vi "Npsv pc test.vi"() -> ()   [LabVIEW 2017]
uses:
  MsgTypeDef.ctl
  <vilib>/WPC Systems Ltd/GECO Driver/Lib/GECOMotion/GECOMotion/_typedefine/Axis Select.ctl
  <vilib>/WPC Systems Ltd/GECO Driver/Lib/GECOMotion/GECOMotion/GECO Motion.lvclass
  <vilib>/WPC Systems Ltd/GECO Driver/Lib/GECOBase/GECO_Driver Class/Motion/_typedefine/GECO_ActiveHighLow.ctl
  <vilib>/WPC Systems Ltd/GECO Driver/Lib/GECOBase/GECO_Driver Class/GECO_Driver.lvclass
  <vilib>/WPC Systems Ltd/GECO Driver/Lib/GECOBase/GECO_Driver Class/Motion/_typedefine/GECO_Motion Operation Mode.ctl
  <vilib>/WPC Systems Ltd/GECO Driver/Lib/GECOBase/GECO_Driver Class/GECO_SlotName.ctl
  <vilib>/WPC Systems Ltd/GECO Driver/Lib/GECOBase/GECO_Driver Class/Motion/_typedefine/GECO_Stepper Output Configuration.ctl
  <vilib>/NI/Modbus Library/API/Modbus API.lvclass
  DataDef.ctl
  GyroDef.ctl
  <vilib>/Instr/_visa.llb/VISA Configure Serial Port (Instr).vi
  Reverse Polarity.ctl
  Forward Polarity.ctl
  Motion Controller Slot.ctl
  Stepper Output Configuration.ctl
  Axis Select.ctl
panel:
  out "RT Program Period":u32
  out "error IO 2":errorcluster
  out "error IO":errorcluster
  out "實際角度":cluster{"A":dbl, "B":dbl}={"A"=-3.299667554384925, "B"=3.520332445615068}
  out "實際角度Chart":cluster{"X":dbl, "Y":dbl}(graph)={"X"=-3.299667554384925, "Y"=3.520332445615068} caption="Waveform Chart - dark"
  out "Gyro\nPeriod":u32
  in  "Main Setting Tab":T1(tab)
  in  "TimerON":bool
  in  "Timer(ms)":i32=1
  in  "Serial Port":refnum<visa-resource-name>="COM3"
  in  "TCP slave port":u32=1
  in  "baud rate":u32=115200
  in  "Byte bits":u32=8
  in  "Modbus Address Starting":u32
  in  "Modbus Number of Inputs":u32=10000
  in  "Resource Name":tag="rio://192.168.0.224/RIO0"
  in  "Servo on":bool
  in  "Axis Select":T2
  in  "Stepper Output Configuration":T3=enum."CW/CCW(Two Pulse)"
  in  "Forward Enable?":bool=TRUE
  in  "Reverse Enable?":bool=TRUE
  in  "Motion Operation Mode":T4(ring)=enum."Velocity"
  in  "Forward Polarity":T5
  in  "Reverse Polarity":T6
  in  "Motion Controller Slot":T7
  in  "Target Position (0)":dbl=10000.0
  in  "Acceleration (100000)":u32=300000
  in  "Velocity (10000)":dbl=100000.0
  in  "Deacceleration (100000)":u32=300000
  in  "PID gains setting Tab":enum32{"Axis 1", "Axis 2", "Axis 3"}(tab)
  in  "PID gains":T8={"proportional gain (Kc)"=0.75, "integral time (Ti, min)"=0.01, "derivative time (Td, min)"=0.0} {"derivative time (Td, min)" format="%#_3f"; "integral time (Ti, min)" format="%#_3f"; "proportional gain (Kc)" format="%#_3f"}
  in  "PID gains 2":T8={"proportional gain (Kc)"=0.75, "integral time (Ti, min)"=0.01, "derivative time (Td, min)"=0.0} {"derivative time (Td, min)" format="%#_3f"; "integral time (Ti, min)" format="%#_3f"; "proportional gain (Kc)" format="%#_3f"}
  in  "PID gains 3":T8={"proportional gain (Kc)"=0.75, "integral time (Ti, min)"=0.01, "derivative time (Td, min)"=0.0} {"derivative time (Td, min)" format="%#_3f"; "integral time (Ti, min)" format="%#_3f"; "proportional gain (Kc)" format="%#_3f"}
  in  "ZABStop":bool
  in  "B":i32
  in  "A":i32
  in  "Z":i32=50
  in  "ZAB Start":bool
  in  "Move Setting":T9
  out "Axis 1":T10
  out "Axis 2":T10
  out "Axis 3":T10
  out "Program Period":u32
  in  "ServoButtonControl":T11
  in  "Connect":bool
  in  "Close":bool
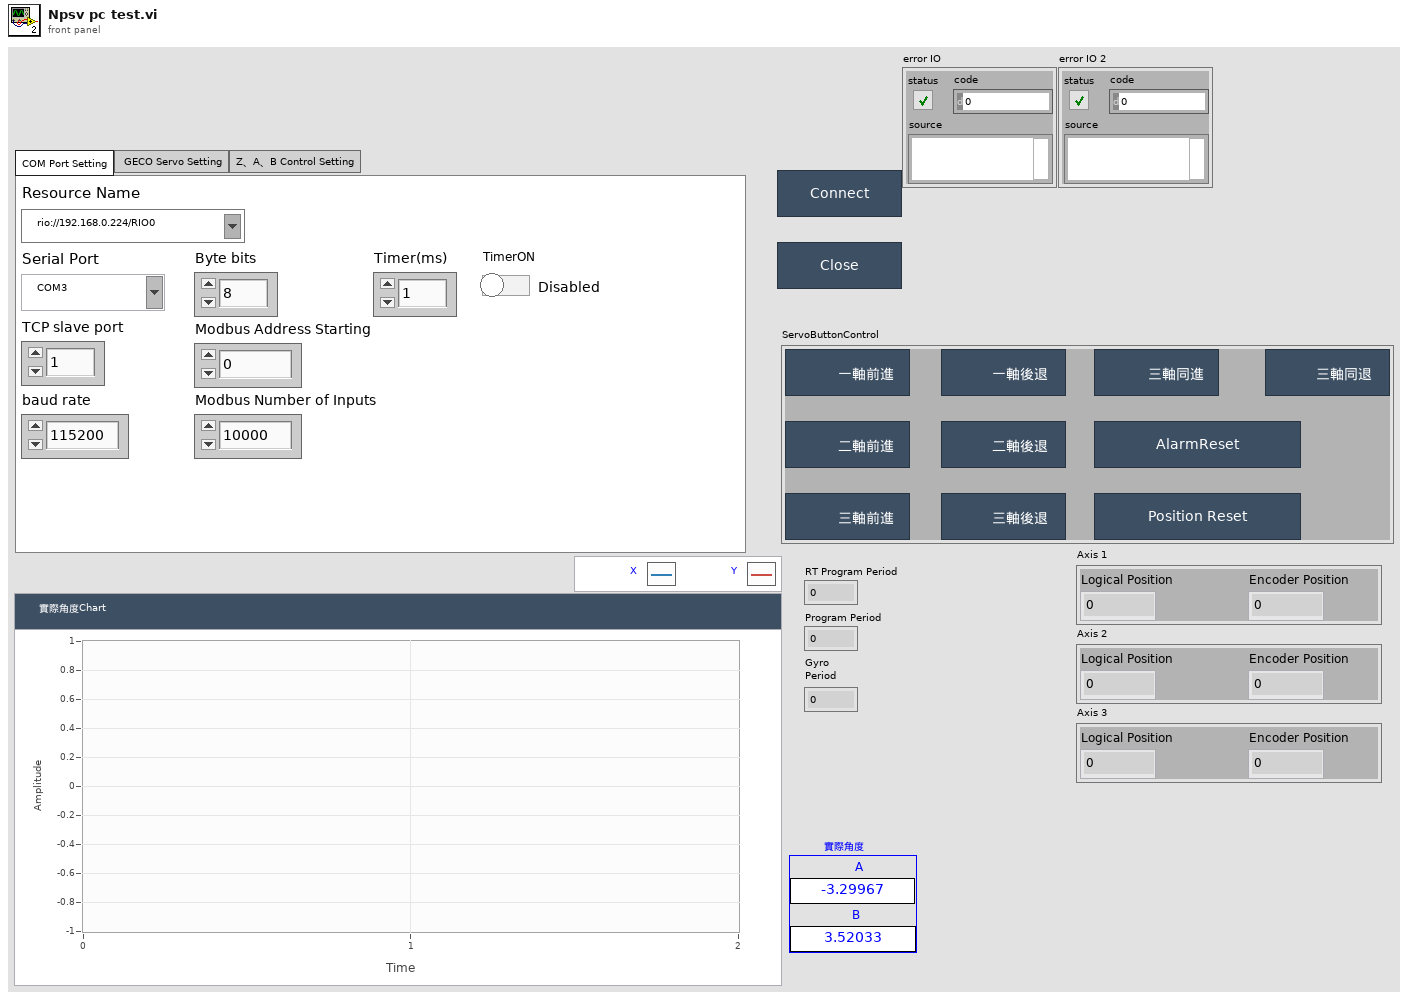
[diagram p1: front panel]
types:
  T1 = enum32{"COM Port Setting", " GECO Servo Setting", "Z、A、B Control Setting"}
  T2 = typedef "Axis Select.ctl" = enum16{"Axis 1", "Axis 2", "Axis 3", "Axis 4"}
  T3 = typedef "Stepper Output Configuration.ctl" = enum16{"Step/Dir(One Pulse)", "CW/CCW(Two Pulse)"}
  T4 = enum16{"Absolute Position", "Relative Position", "Velocity"}
  T5 = typedef "Forward Polarity.ctl" = enum16{"Active High", "Active Low"}
  T6 = typedef "Reverse Polarity.ctl" = enum16{"Active High", "Active Low"}
  T7 = typedef "Motion Controller Slot.ctl" = enum16{"C1", "C2", "C3", "C4"}
  T8 = cluster{"proportional gain (Kc)":dbl, "integral time (Ti, min)":dbl, "derivative time (Td, min)":dbl}
  T9 = typedef "軌跡設定.ctl" = u16
  T10 = cluster{"Encoder Position":i32, "Logical Position":i32}
  T11 = cluster{"三軸同退":bool, "三軸同進":bool, "三軸後退":bool, "三軸前進":bool, "二軸後退":bool, "二軸前進":bool, "一軸後退":bool, "一軸前進":bool, "Reset Encoder Position":bool, "AlarmReset":bool}
  T12 = typedef "GyroDef.ctl" = cluster{"Byte bits":u16, "baud rate":u32, "實際角度":cluster{"A":dbl, "B":dbl}, "COM Port":refnum<visa-resource-name>, "Save Path":refnum<file>}
  T13 = typedef "DataDef.ctl" = cluster{"address starting":u16, "狀態":enum16{"初始化", "讀取", "寫入", "停止"}, "理想角度":cluster{"A":dbl, "B":dbl}, "register values":i16[], "Modbus COM":refnum<class "Modbus API.lvclass">, "TCP slave port":u16, " baud rate":u32, "Byte bits":u16, "ServoButtonControl":cluster{"三軸同退":bool, "三軸同進":bool, "三軸後退":bool, "三軸前進":bool, "二軸後退":bool, "二軸前進":bool, "一軸後退":bool, "一軸前進":bool}, "Serial Number":string, "GECO_Driver out":refnum<class "GECO_Driver.lvclass">, "number of inputs":u16, "ServoSetting":cluster{"Axis Select":T14, "Stepper Output Configuration":T15, "Motion Operation Mode":T16, "Motion Controller Slot":T17, "Singel Axis Move Paramters":cluster{"Motion Operation Mode":T16, "Target Position (0)":i32, "Velocity (10000)":i32, "Acceleration (100000)":u32, "Deacceleration (100000)":u32}, "Reverse":cluster{"Reverse Enable":bool, "Reverse Polarity":T18}, "Forward":cluster{"Forward Enable":bool, "Forward Polarity":T18}}, "GECO Motion out":refnum<class "GECO Motion.lvclass">, "Servo on":bool, "Axis 1 Position":cluster{"Encoder Position":i32, "Logical Position":i32}, "Axis 2 Position":cluster{"Encoder Position":i32, "Logical Position":i32}, "Axis 3 Position":cluster{"Encoder Position":i32, "Logical Position":i32}, "PIDSetting":cluster{"Z":i32, "A":i32, "B":i32, "Move Setting":T19, "Axis Pulse":dbl, "Axis Length":dbl, "PID gains ":cluster{"proportional gain (Kc)":dbl, "integral time (Ti, min)":dbl, "derivative time (Td, min)":dbl}}, "resource name":tag, "Save Path":refnum<file>}
  T14 = typedef "GECO Motion.lvclass/Axis Select.ctl" = enum16{"Axis 1", "Axis 2", "Axis 3", "Axis 4"}
  T15 = typedef "GECO_Driver.lvclass/GECO_Stepper Output Configuration.ctl" = enum16{"Step/Dir(One Pulse)", "CW/CCW(Two Pulse)"}
  T16 = typedef "GECO_Driver.lvclass/GECO_Motion Operation Mode.ctl" = enum16{"Absolute Position", "Relative Position", "Velocity"}
  T17 = typedef "GECO_Driver.lvclass/GECO_SlotName.ctl" = enum16{"C1", "C2", "C3", "C4"}
  T18 = typedef "GECO_Driver.lvclass/GECO_ActiveHighLow.ctl" = enum16{"Active High", "Active Low"}
  T19 = typedef "­y¸ñ.ctl" = u16
  T20 = typedef "MsgTypeDef.ctl" = cluster{"CMD":string, "DATA":variant}
  T21 = enum16{"open", "replace", "create", "open or create", "replace or create", "replace or create with confirmation"}
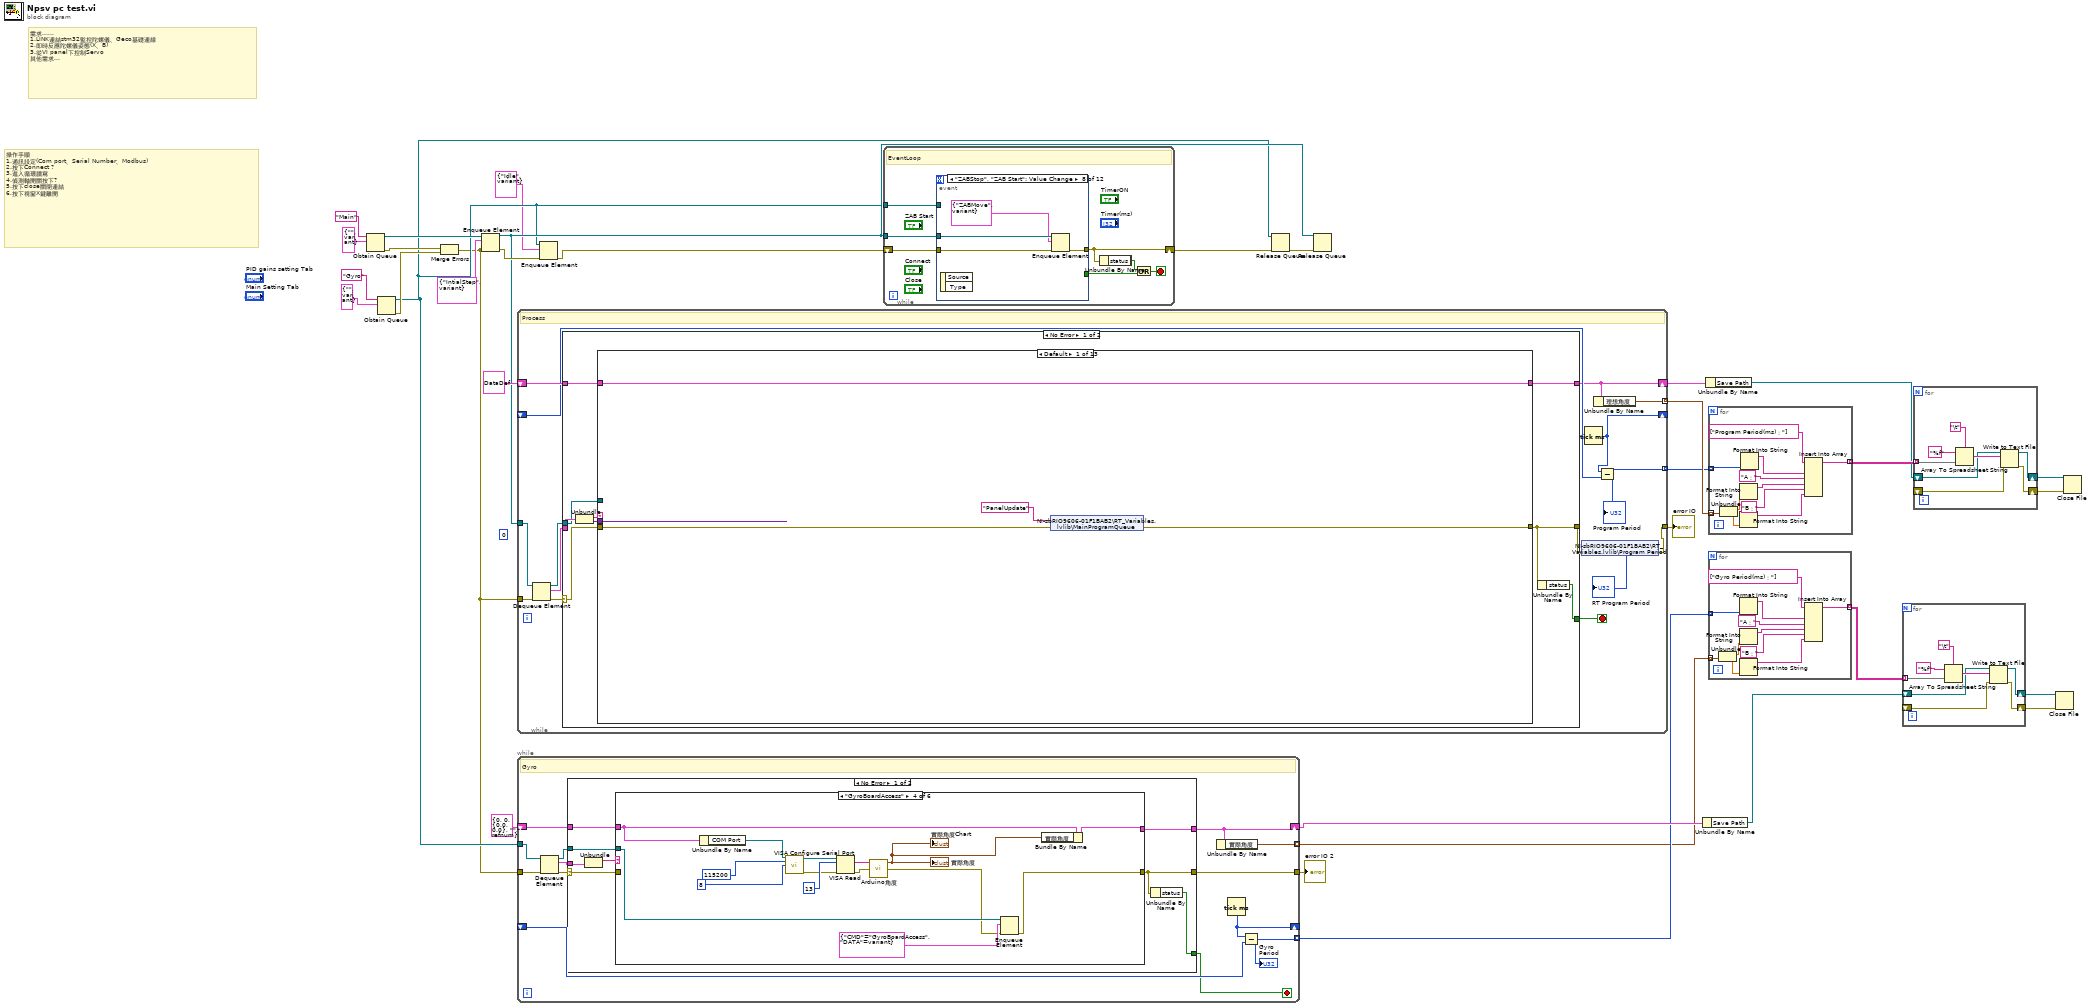
[diagram p0: block diagram]
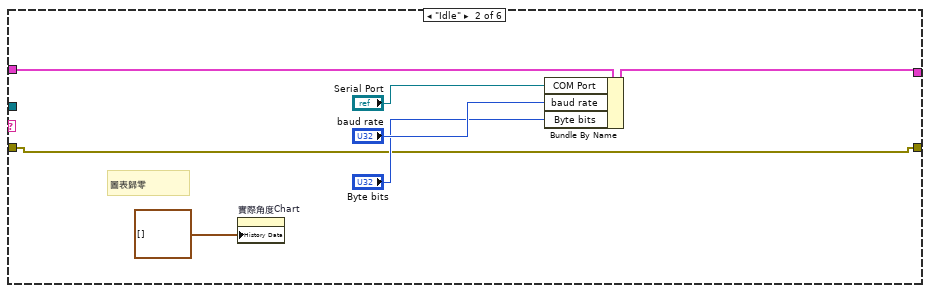
[diagram p3: hidden frame]
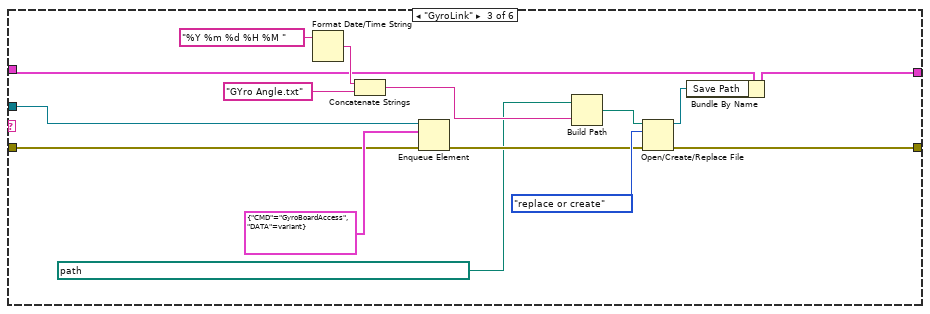
[diagram p4: hidden frame]
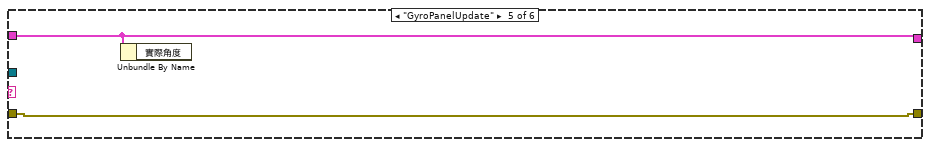
[diagram p5: hidden frame]
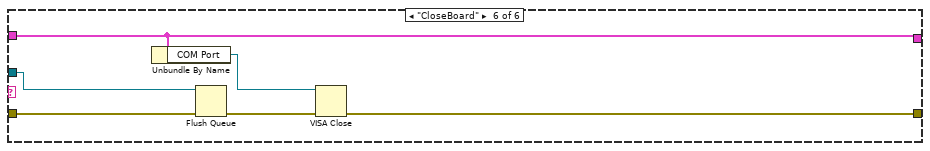
[diagram p6: hidden frame]
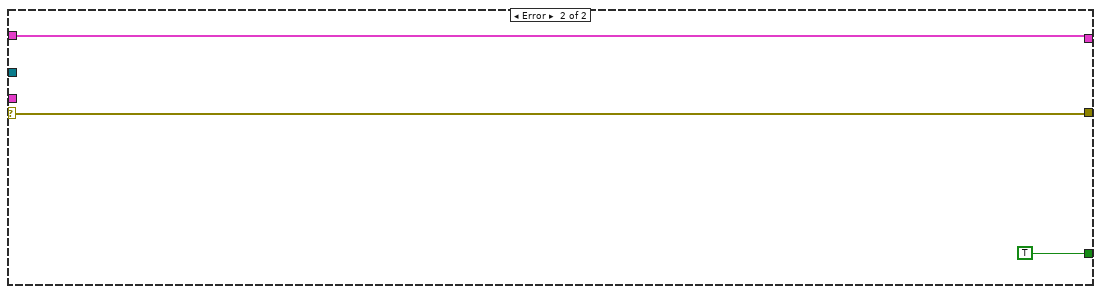
[diagram p7: hidden frame]
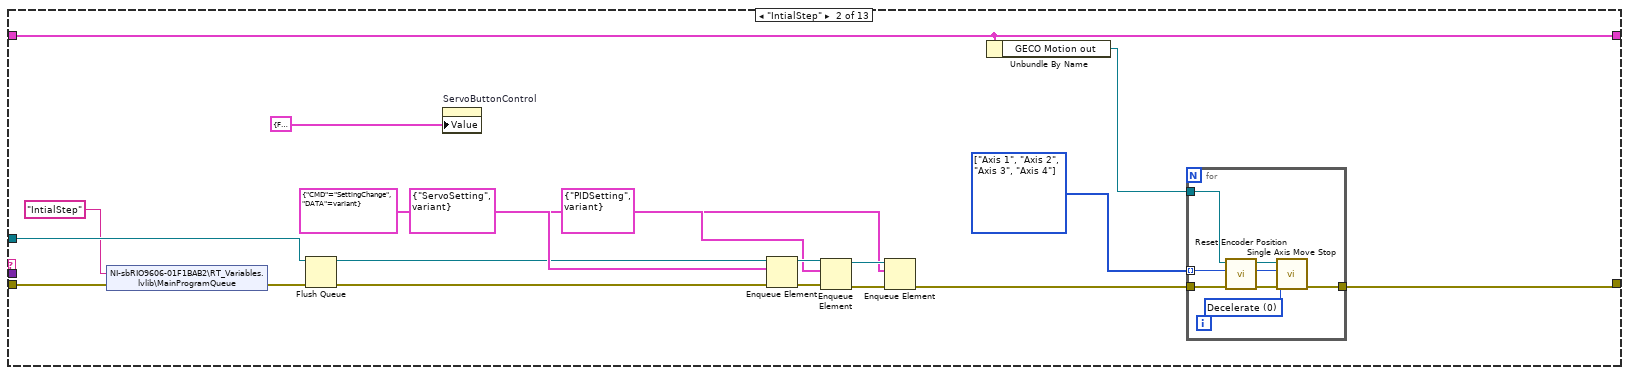
[diagram p8: hidden frame]
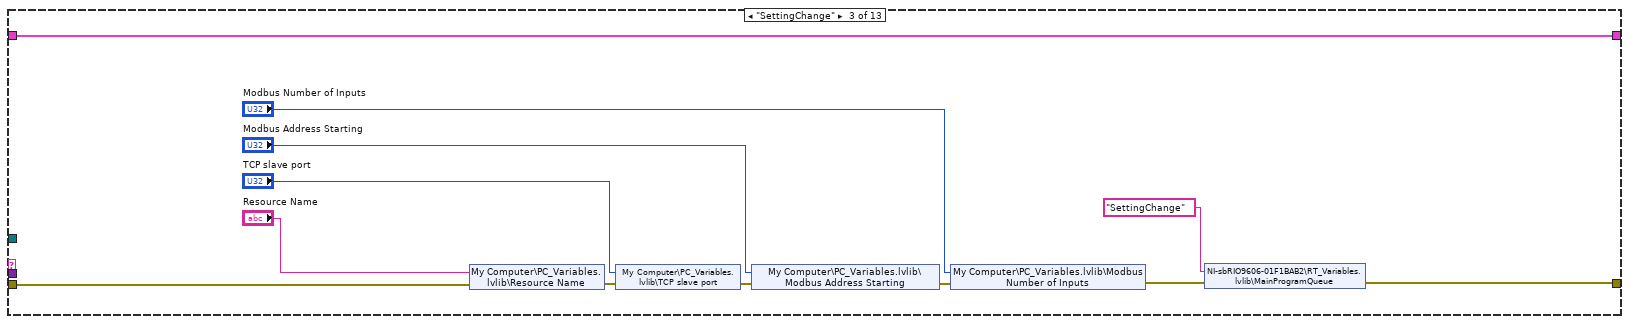
[diagram p9: hidden frame]
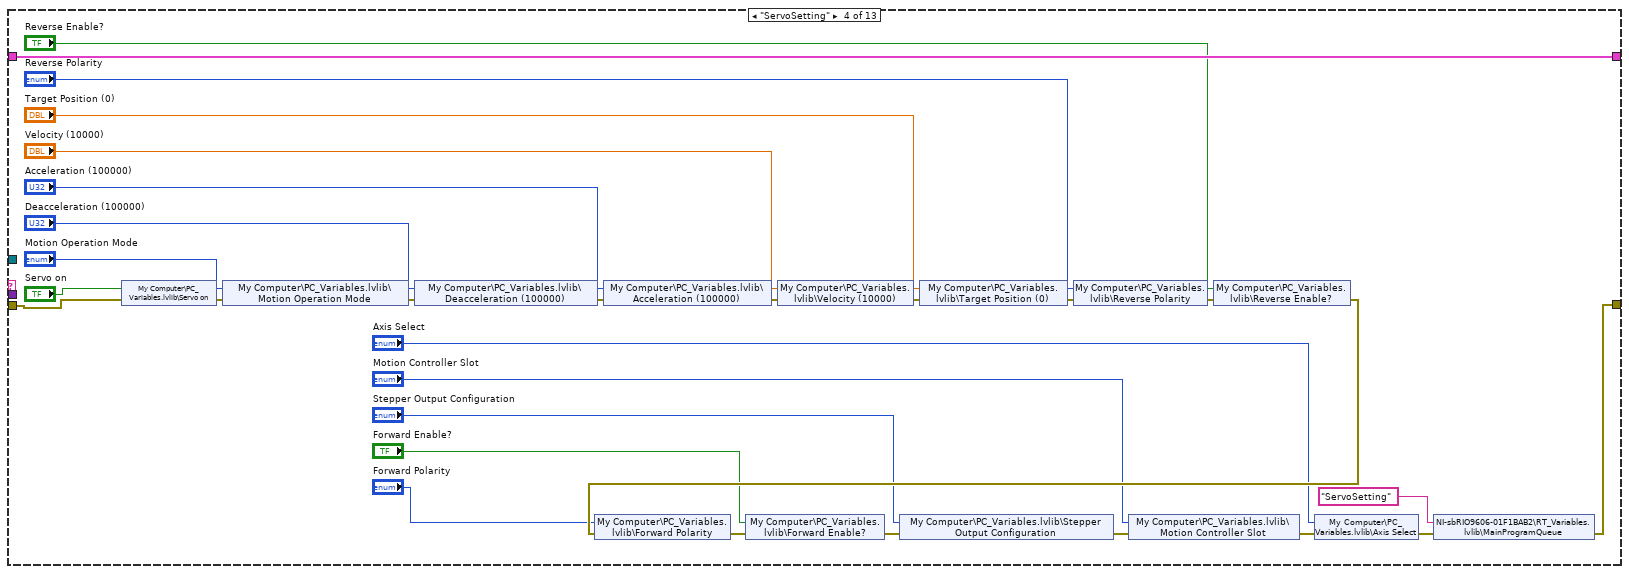
[diagram p10: hidden frame]
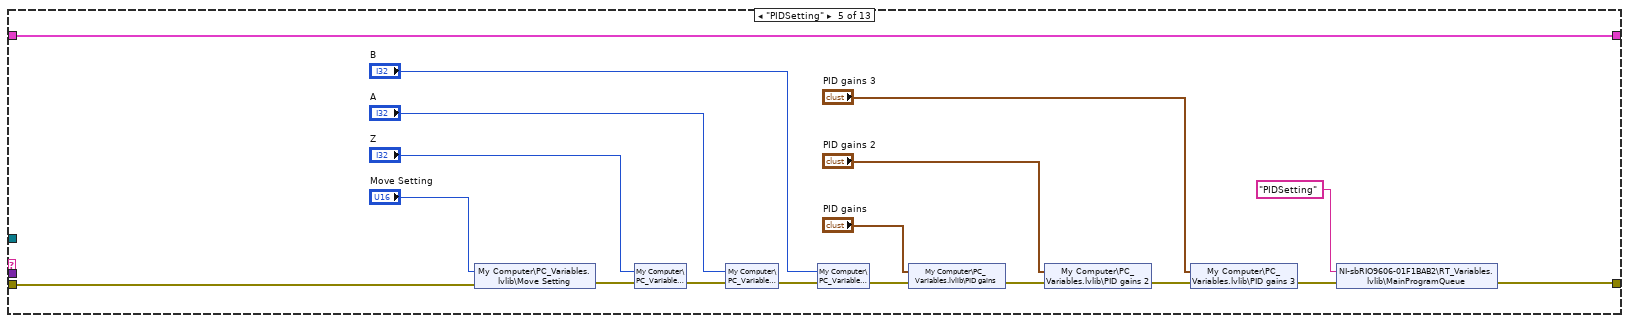
[diagram p11: hidden frame]
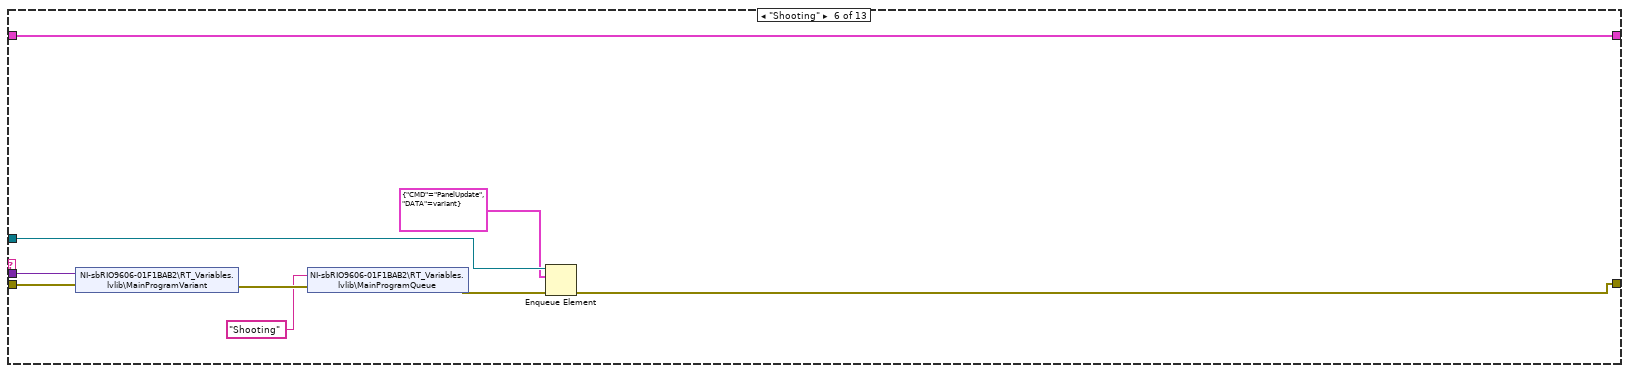
[diagram p12: hidden frame]
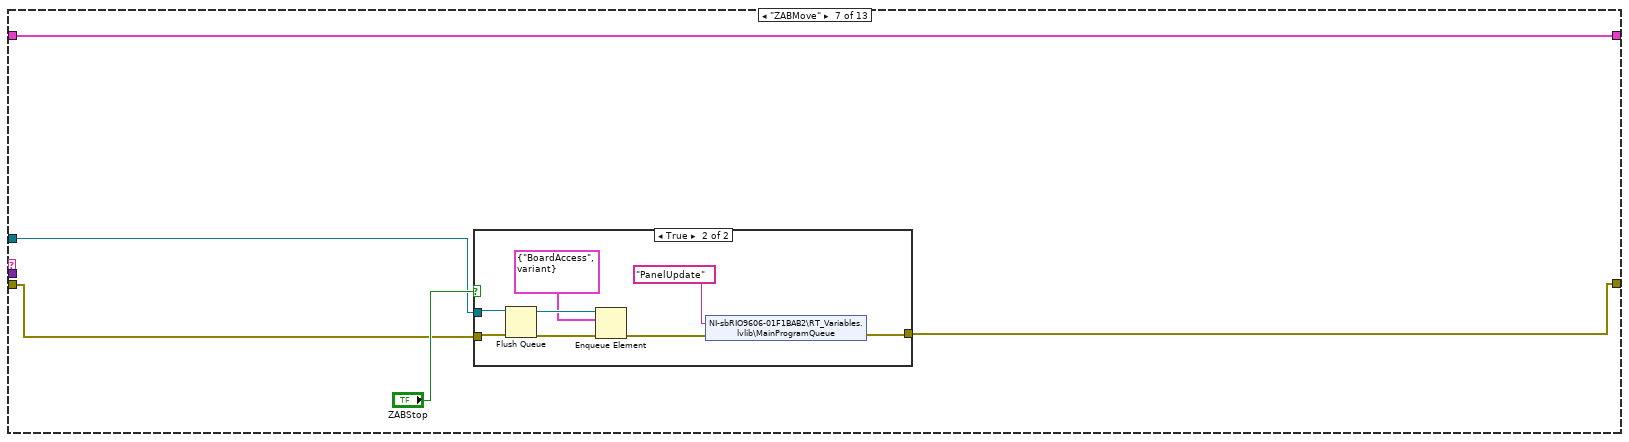
[diagram p13: hidden frame]
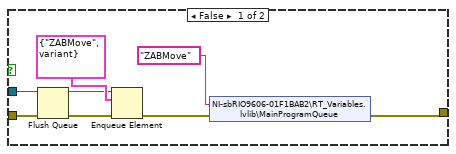
[diagram p14: hidden frame]
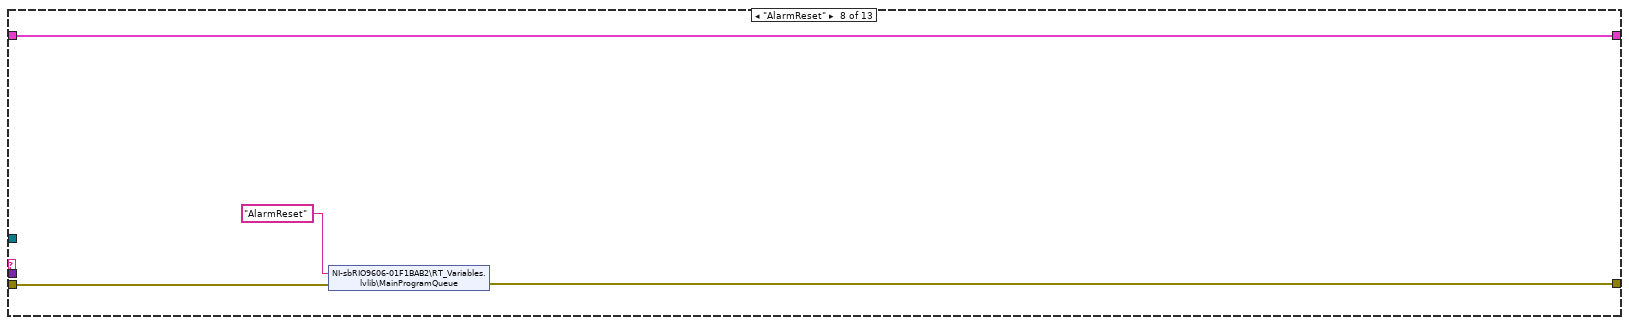
[diagram p15: hidden frame]
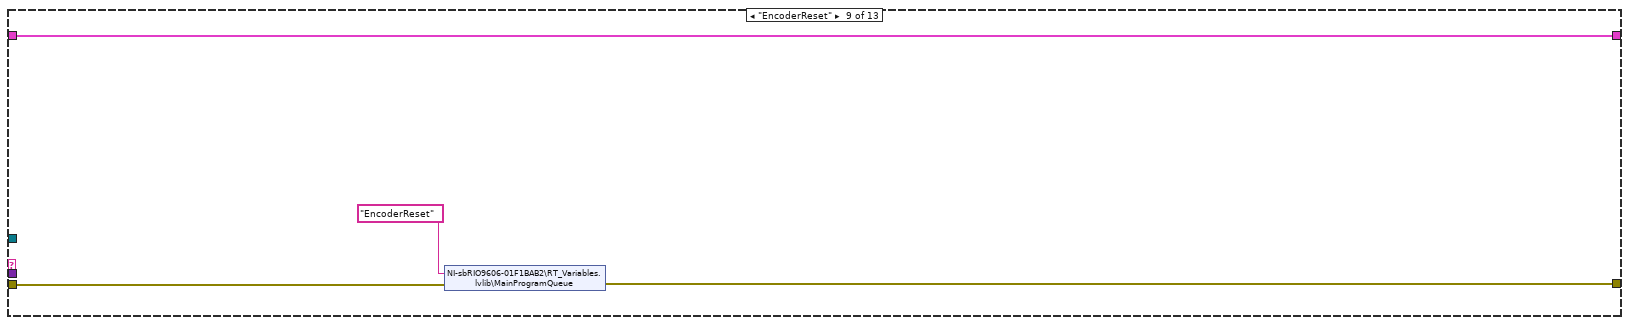
[diagram p16: hidden frame]
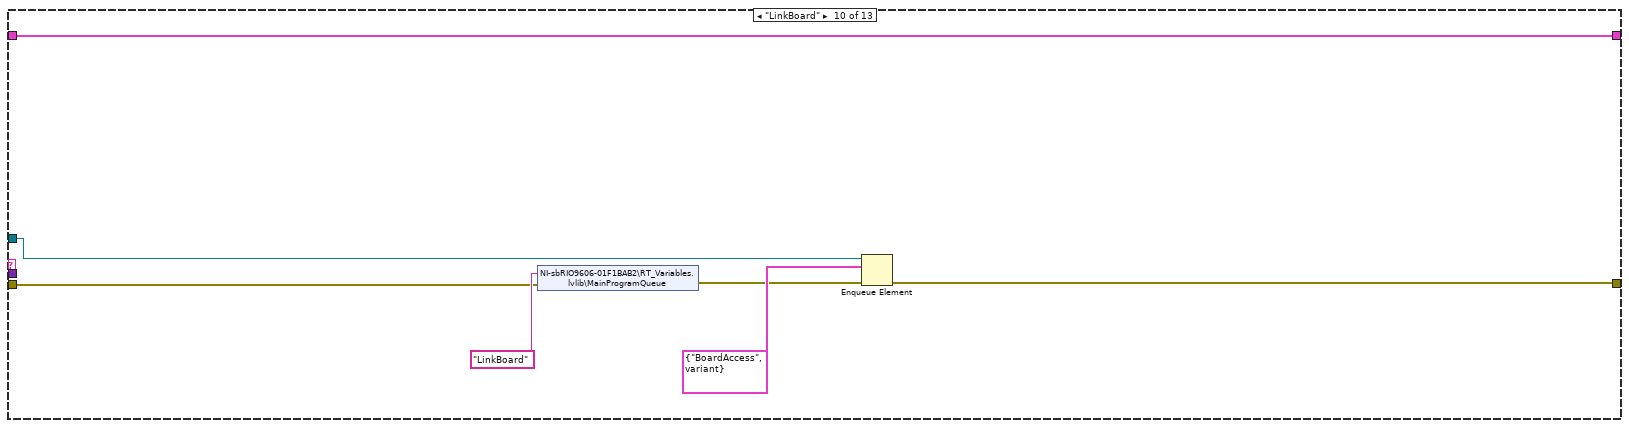
[diagram p17: hidden frame]
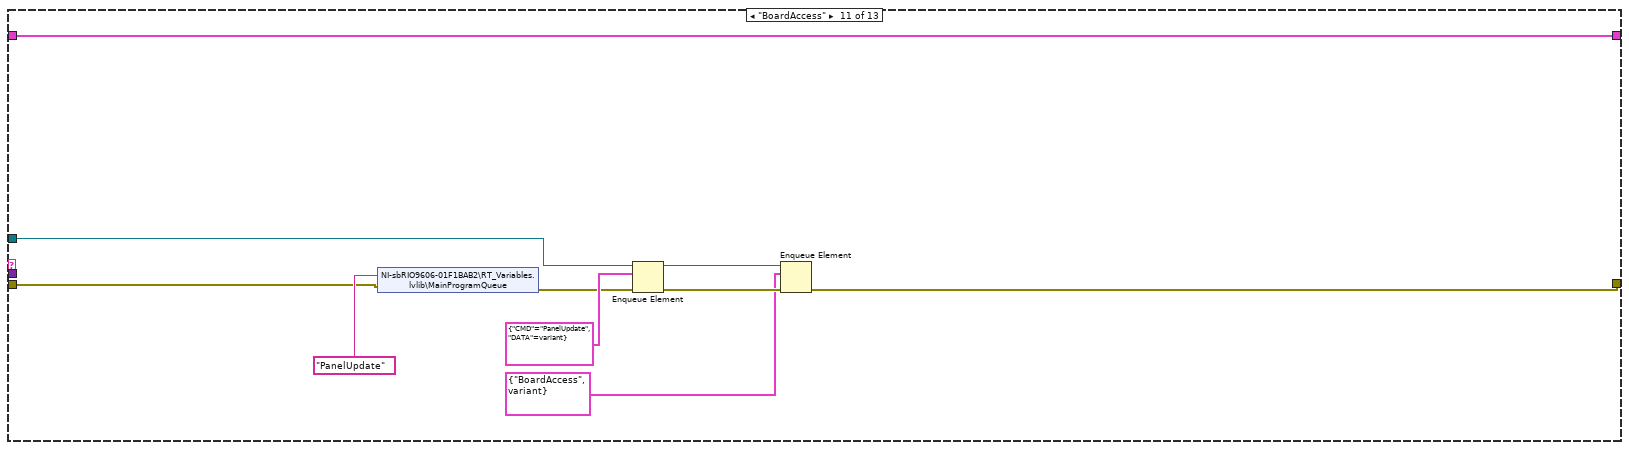
[diagram p18: hidden frame]
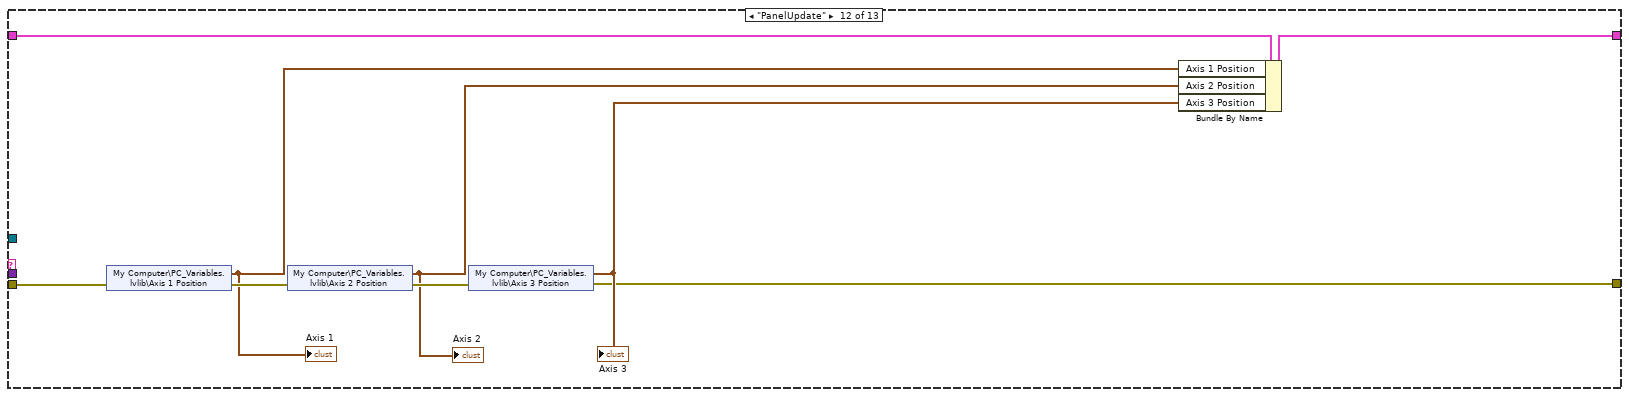
[diagram p19: hidden frame]
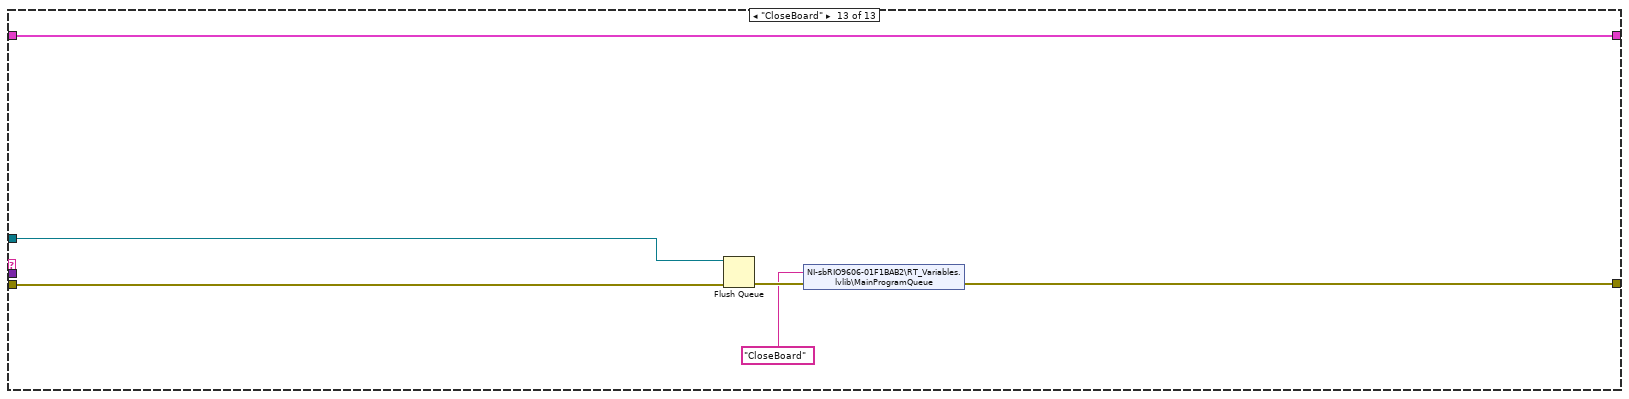
[diagram p20: hidden frame]
diagram:
  (unwired) 0
  # "操作手順\n1.通訊設定(Com port、Serial Number、Modbus)\n2.按下Connect ?\n3.進入循環讀寫\n4.偵測軸開關按下?\n5.按下close關閉連結\n6.按下視窗X鍵離開"
  # "需求......\n1.LINK連結stm32監控陀螺儀、Geco基礎連線\n2.即時反應陀螺儀姿態(X、B)\n3.從VI panel下控制Servo\n其他需求..."
  n1 = Obtain Queue(name (unnamed)="Main", element data type=T20 {"CMD"="", "DATA"=variant}) -> (queue out=w30:refnum<queue>, error out=w25:errorcluster)  [unwired: 3 in, 1 out]
  n2 = Obtain Queue(name (unnamed)="Gyro", element data type=T20 {"CMD"="", "DATA"=variant}) -> (queue out=w20:refnum<queue>, error out=w26:errorcluster)  [unwired: 3 in, 1 out]
  n3 = Merge Errors(w25, w26) -> (w18:errorcluster)
  n4 = Enqueue Element(queue=w30, element=T20 {"CMD"="IntialStep", "DATA"=variant}, error in (no error)=w18) -> (queue out=w21:refnum<queue>, error out=w23:errorcluster)  [unwired: 1 in, 1 out]
  n5 = while {
    tunnel: w21 -> [w49]
    shift-right: [w40] -> w13
    shift-left: T13 {"address starting"=0, "狀態"=enum."初始化", "理想角度"={"A"=0.0, "B"=0.0}, "register values"=[], "Modbus COM"=refnum, "TCP slave port"=1, " baud rate"=0, "Byte bits"=0, "ServoButtonControl"={"三軸同退"=FALSE, "三軸同進"=FALSE, "三軸後退"=FALSE, "三軸前進"=FALSE, "二軸後退"=FALSE, "二軸前進"=FALSE, "一軸後退"=FALSE, "一軸前進"=FALSE}, "Serial Number"="", "GECO_Driver out"=refnum, "number of inputs"=0, "ServoSetting"={"Axis Select"=enum."Axis 1", "Stepper Output Configuration"=enum."Step/Dir(One Pulse)", "Motion Operation Mode"=enum."Absolute Position", "Motion Controller Slot"=enum."C1", "Singel Axis Move Paramters"={"Motion Operation Mode"=enum."Velocity", "Target Position (0)"=10000, "Velocity (10000)"=1, "Acceleration (100000)"=100000, "Deacceleration (100000)"=1}, "Reverse"={"Reverse Enable"=FALSE, "Reverse Polarity"=enum."Active Low"}, "Forward"={"Forward Enable"=FALSE, "Forward Polarity"=enum."Active Low"}}, "GECO Motion out"=refnum, "Servo on"=FALSE, "Axis 1 Position"={"Encoder Position"=0, "Logical Position"=0}, "Axis 2 Position"={"Encoder Position"=0, "Logical Position"=0}, "Axis 3 Position"={"Encoder Position"=0, "Logical Position"=0}, "PIDSetting"={"Z"=10000, "A"=10000, "B"=10000, "Move Setting"=1, "Axis Pulse"=10000.0, "Axis Length"=10000.0, "PID gains "={"proportional gain (Kc)"=1.0, "integral time (Ti, min)"=0.01, "derivative time (Td, min)"=0.0}}, "resource name"="", "Save Path"=refnum} -> [w45]
    tunnel: w18 -> [w43]
    shift-right: [w42] -> _
    shift-left: _ -> [w41]
    tunnel: [w39] -> w16 mode=indexing
    tunnel: [w38] -> w15 mode=indexing
    tunnel: [w36] -> w2
    stop <- w46 stop-if-true
    # "Process"
    n6 = Dequeue Element(queue=w49, error in (no error)=w43) -> (queue out=w44:refnum<queue>, element=w47:T20, error out=w48:errorcluster)  [unwired: 1 in, 1 out]
    n7 = case shown="No Error" w48 {
      selector: w48 -> [w54 w220]
      tunnel: w47 -> [w58 _]
      tunnel: [w51 TRUE] -> w46
      tunnel: [w56 w221] -> w40
      tunnel: w45 -> [w55 w221]
      tunnel: w44 -> [w53 _]
      tunnel: [w50 w220] -> w37
      frame No Error {
        n8 = Unbundle(w58) -> ("CMD"=w57:string, "DATA"=w52:variant)
        n9 = case shown="Default" w57 {
          tunnel: [w62 w66 w100 w131 w149 w158 w159 w183 w187 w191 w198 w212 w219] -> w56
          tunnel: w55 -> [w62 w66 w100 w131 w149 w158 w159 w183 w187 w191 w198 w213 w219]
          tunnel: w54 -> [w61 w64 w99 w130 w148 w156 w161 w182 w185 w189 w196 w209 w217]
          tunnel: [w60 w76 w98 w103 w144 w151 w160 w180 w184 w194 w201 w205 w215] -> w50
          tunnel: w53 -> [_ w70 _ _ _ w152 w162 _ _ w192 w204 _ w218]
          tunnel: w52 -> [_ _ _ _ _ w157 _ _ _ _ _ _ _]
          frame Default {
            n10 = shared-variable "NI-sbRIO9606-01F1BAB2\\RT_Variables.lvlib\\MainProgramQueue"("PanelUpdate", error in=w61) -> (error out=w60:errorcluster)
          }
          frame "IntialStep" {
            w74 = T14[] [enum."Axis 1", enum."Axis 2", enum."Axis 3", enum."Axis 4"] items=["Axis 1", "Axis 2", "Axis 3", "Axis 4"]
            n11 = shared-variable "NI-sbRIO9606-01F1BAB2\\RT_Variables.lvlib\\MainProgramQueue"("IntialStep" ("CMD"), error in=w64) -> (error out=w65:errorcluster)
            n12 = Flush Queue(queue=w70, error in (no error)=w65) -> (queue out=w69:refnum<queue>, error out=w68:errorcluster)  [unwired: 1 out]
            n13 = property on="ServoButtonControl" class="Clust"("Value"=T11 {"三軸同退"=FALSE, "三軸同進"=FALSE, "三軸後退"=FALSE, "三軸前進"=FALSE, "二軸後退"=FALSE, "二軸前進"=FALSE, "一軸後退"=FALSE, "一軸前進"=FALSE, "Reset Encoder Position"=FALSE, "AlarmReset"=FALSE} ("ServoButtonControl")) -> ()  [unwired: 2 in, 2 out]
            n14 = Enqueue Element(queue=w69, element=T20 {"CMD"="SettingChange", "DATA"=variant}, error in (no error)=w68) -> (queue out=w79:refnum<queue>, error out=w80:errorcluster)  [unwired: 1 in, 1 out]
            n15 = Enqueue Element(queue=w79, element=T20 {"CMD"="ServoSetting", "DATA"=variant}, error in (no error)=w80) -> (queue out=w73:refnum<queue>, error out=w72:errorcluster)  [unwired: 1 in, 1 out]
            n16 = Enqueue Element(queue=w73, element=T20 {"CMD"="PIDSetting", "DATA"=variant}, error in (no error)=w72) -> (error out=w67:errorcluster)  [unwired: 1 in, 2 out]
            n17 = Unbundle By Name(w66) -> ("GECO Motion out"=w75:refnum<class "GECO Motion.lvclass">)
            n18 = for {
              tunnel: w67 -> [w89]
              tunnel: [w83] -> w76
              tunnel: w75 -> [w88]
              tunnel: w74 -> [w87] mode=indexing
              w82 = u16 0 items=["Decelerate", "Halt"] ("Motion Stop Type")
              n19 = call <vilib>:"Reset Encoder Position.vi"("error in (no error)"=w89, "Axis Select"=w87, "GECO Motion in"=w88) -> ("error out"=w86:errorcluster, "Axis Select out"=w85:T14, "GECO Motion out"=w84:refnum<class "GECO Motion.lvclass">)  [unwired: 6 in]
              n20 = call <vilib>:"Single Axis Move Stop.vi"("error in (no error)"=w86, "Motion Stop Type"=w82, "Axis Select"=w85, "GECO Motion in"=w84) -> ("error out"=w83:errorcluster)  [unwired: 5 in, 2 out]
            }
          }
          frame "SettingChange" {
            n21 = shared-variable "My Computer\\PC_Variables.lvlib\\Resource Name"("Resource Name", error in=w99) -> (error out=w97:errorcluster)
            n22 = shared-variable "My Computer\\PC_Variables.lvlib\\TCP slave port"("TCP slave port", error in=w97) -> (error out=w96:errorcluster)
            n23 = shared-variable "My Computer\\PC_Variables.lvlib\\Modbus Address Starting"("Modbus Address Starting", error in=w96) -> (error out=w95:errorcluster)
            n24 = shared-variable "My Computer\\PC_Variables.lvlib\\Modbus Number of Inputs"("Modbus Number of Inputs", error in=w95) -> (error out=w94:errorcluster)
            n25 = shared-variable "NI-sbRIO9606-01F1BAB2\\RT_Variables.lvlib\\MainProgramQueue"("SettingChange" ("CMD"), error in=w94) -> (error out=w98:errorcluster)
          }
          frame "ServoSetting" {
            n26 = shared-variable "My Computer\\PC_Variables.lvlib\\Servo on"("Servo on", error in=w130) -> (error out=w128:errorcluster)
            n27 = shared-variable "My Computer\\PC_Variables.lvlib\\Motion Operation Mode"("Motion Operation Mode", error in=w128) -> (error out=w127:errorcluster)
            n28 = shared-variable "My Computer\\PC_Variables.lvlib\\Deacceleration (100000)"("Deacceleration (100000)", error in=w127) -> (error out=w126:errorcluster)
            n29 = shared-variable "My Computer\\PC_Variables.lvlib\\Acceleration (100000)"("Acceleration (100000)", error in=w126) -> (error out=w125:errorcluster)
            n30 = shared-variable "My Computer\\PC_Variables.lvlib\\Velocity (10000)"("Velocity (10000)", error in=w125) -> (error out=w124:errorcluster)
            n31 = shared-variable "My Computer\\PC_Variables.lvlib\\Target Position (0)"("Target Position (0)", error in=w124) -> (error out=w123:errorcluster)
            n32 = shared-variable "My Computer\\PC_Variables.lvlib\\Reverse Polarity"("Reverse Polarity", error in=w123) -> (error out=w122:errorcluster)
            n33 = shared-variable "My Computer\\PC_Variables.lvlib\\Reverse Enable?"("Reverse Enable?", error in=w122) -> (error out=w129:errorcluster)
            n34 = shared-variable "My Computer\\PC_Variables.lvlib\\Forward Polarity"("Forward Polarity", error in=w129) -> (error out=w113:errorcluster)
            n35 = shared-variable "My Computer\\PC_Variables.lvlib\\Forward Enable?"("Forward Enable?", error in=w113) -> (error out=w112:errorcluster)
            n36 = shared-variable "My Computer\\PC_Variables.lvlib\\Stepper Output Configuration"("Stepper Output Configuration", error in=w112) -> (error out=w111:errorcluster)
            n37 = shared-variable "My Computer\\PC_Variables.lvlib\\Motion Controller Slot"("Motion Controller Slot", error in=w111) -> (error out=w110:errorcluster)
            n38 = shared-variable "My Computer\\PC_Variables.lvlib\\Axis Select"("Axis Select", error in=w110) -> (error out=w104:errorcluster)
            n39 = shared-variable "NI-sbRIO9606-01F1BAB2\\RT_Variables.lvlib\\MainProgramQueue"("ServoSetting" ("CMD"), error in=w104) -> (error out=w103:errorcluster)
          }
          frame "PIDSetting" {
            n40 = shared-variable "My Computer\\PC_Variables.lvlib\\Move Setting"("Move Setting", error in=w148) -> (error out=w147:errorcluster)
            n41 = shared-variable "My Computer\\PC_Variables.lvlib\\Z"("Z", error in=w147) -> (error out=w146:errorcluster)
            n42 = shared-variable "My Computer\\PC_Variables.lvlib\\A"("A", error in=w146) -> (error out=w145:errorcluster)
            n43 = shared-variable "My Computer\\PC_Variables.lvlib\\B"("B", error in=w145) -> (error out=w135:errorcluster)
            n44 = shared-variable "My Computer\\PC_Variables.lvlib\\PID gains"("PID gains", error in=w135) -> (error out=w134:errorcluster)
            n45 = shared-variable "My Computer\\PC_Variables.lvlib\\PID gains 2"("PID gains 2", error in=w134) -> (error out=w133:errorcluster)
            n46 = shared-variable "My Computer\\PC_Variables.lvlib\\PID gains 3"("PID gains 3", error in=w133) -> (error out=w132:errorcluster)
            n47 = shared-variable "NI-sbRIO9606-01F1BAB2\\RT_Variables.lvlib\\MainProgramQueue"("PIDSetting", error in=w132) -> (error out=w144:errorcluster)
          }
          frame "Shooting" {
            n48 = shared-variable "NI-sbRIO9606-01F1BAB2\\RT_Variables.lvlib\\MainProgramVariant"(w157, error in=w156) -> (error out=w155:errorcluster)
            n49 = shared-variable "NI-sbRIO9606-01F1BAB2\\RT_Variables.lvlib\\MainProgramQueue"("Shooting" ("CMD"), error in=w155) -> (error out=w153:errorcluster)
            n50 = Enqueue Element(queue=w152, element=T20 {"CMD"="PanelUpdate", "DATA"=variant}, error in (no error)=w153) -> (error out=w151:errorcluster)  [unwired: 1 in, 2 out]
          }
          frame "ZABMove" {
            n51 = case shown="True" "ZABStop" {
              tunnel: [w165 w173] -> w160
              tunnel: w162 -> [w168 w176]
              tunnel: w161 -> [w167 w175]
              frame False {
                n52 = Flush Queue(queue=w168, error in (no error)=w167) -> (queue out=w169:refnum<queue>, error out=w170:errorcluster)  [unwired: 1 out]
                n53 = Enqueue Element(queue=w169, element=T20 {"CMD"="ZABMove", "DATA"=variant}, error in (no error)=w170) -> (error out=w166:errorcluster)  [unwired: 1 in, 2 out]
                n54 = shared-variable "NI-sbRIO9606-01F1BAB2\\RT_Variables.lvlib\\MainProgramQueue"("ZABMove" ("CMD"), error in=w166) -> (error out=w165:errorcluster)
              }
              frame True {
                n55 = Flush Queue(queue=w176, error in (no error)=w175) -> (queue out=w179:refnum<queue>, error out=w178:errorcluster)  [unwired: 1 out]
                n56 = Enqueue Element(queue=w179, element=T20 {"CMD"="BoardAccess", "DATA"=variant}, error in (no error)=w178) -> (error out=w172:errorcluster)  [unwired: 1 in, 2 out]
                n57 = shared-variable "NI-sbRIO9606-01F1BAB2\\RT_Variables.lvlib\\MainProgramQueue"("PanelUpdate" ("CMD"), error in=w172) -> (error out=w173:errorcluster)
              }
            }
          }
          frame "AlarmReset" {
            n58 = shared-variable "NI-sbRIO9606-01F1BAB2\\RT_Variables.lvlib\\MainProgramQueue"("AlarmReset", error in=w182) -> (error out=w180:errorcluster)
          }
          frame "EncoderReset" {
            n59 = shared-variable "NI-sbRIO9606-01F1BAB2\\RT_Variables.lvlib\\MainProgramQueue"("EncoderReset", error in=w185) -> (error out=w184:errorcluster)
          }
          frame "LinkBoard" {
            n60 = shared-variable "NI-sbRIO9606-01F1BAB2\\RT_Variables.lvlib\\MainProgramQueue"("LinkBoard", error in=w189) -> (error out=w188:errorcluster)
            n61 = Enqueue Element(queue=w192, element=T20 {"CMD"="BoardAccess", "DATA"=variant}, error in (no error)=w188) -> (error out=w194:errorcluster)  [unwired: 1 in, 2 out]
          }
          frame "BoardAccess" {
            n62 = shared-variable "NI-sbRIO9606-01F1BAB2\\RT_Variables.lvlib\\MainProgramQueue"("PanelUpdate", error in=w196) -> (error out=w195:errorcluster)
            n63 = Enqueue Element(queue=w204, element=T20 {"CMD"="PanelUpdate", "DATA"=variant}, error in (no error)=w195) -> (queue out=w203:refnum<queue>, error out=w202:errorcluster)  [unwired: 1 in, 1 out]
            n64 = Enqueue Element(queue=w203, element=T20 {"CMD"="BoardAccess", "DATA"=variant}, error in (no error)=w202) -> (error out=w201:errorcluster)  [unwired: 1 in, 2 out]
          }
          frame "PanelUpdate" {
            n65 = shared-variable "My Computer\\PC_Variables.lvlib\\Axis 1 Position"(error in=w209) -> (w208:T10, error out=w211:errorcluster)
            "Axis 1" <- w208
            n66 = shared-variable "My Computer\\PC_Variables.lvlib\\Axis 2 Position"(error in=w211) -> (w207:T10, error out=w210:errorcluster)
            "Axis 2" <- w207
            n67 = shared-variable "My Computer\\PC_Variables.lvlib\\Axis 3 Position"(error in=w210) -> (w206:T10, error out=w205:errorcluster)
            "Axis 3" <- w206
            n68 = Bundle By Name(cluster=w213, "Axis 1 Position"=w208, "Axis 2 Position"=w207, "Axis 3 Position"=w206) -> (w212:T13)
          }
          frame "CloseBoard" {
            n69 = Flush Queue(queue=w218, error in (no error)=w217) -> (error out=w216:errorcluster)  [unwired: 2 out]
            n70 = shared-variable "NI-sbRIO9606-01F1BAB2\\RT_Variables.lvlib\\MainProgramQueue"("CloseBoard", error in=w216) -> (error out=w215:errorcluster)
          }
        }
        n71 = Unbundle By Name(w50) -> ("status"=w51:bool)
      }
      frame Error {
      }
    }
    n72 = shared-variable "NI-sbRIO9606-01F1BAB2\\RT_Variables.lvlib\\Program Period"(error in=w37) -> (→"RT Program Period":u32, error out=w36:errorcluster)
    n73 = Tick Count (ms)() -> (millisecond timer value=w42:u32)
    n74 = Unbundle By Name(w40) -> ("理想角度"=w39:cluster{"A":dbl, "B":dbl})
    n75 = Subtract(x=w42, y=w41) -> (x-y=w38:u32)
    "Program Period" <- w38
  }
  "error IO" <- w2
  n76 = while {
    tunnel: w20 -> [w235]
    tunnel: w18 -> [w234]
    shift-right: [w229] -> w11
    shift-left: T12 {"Byte bits"=0, "baud rate"=0, "實際角度"={"A"=0.0, "B"=0.0}, "COM Port"="", "Save Path"=refnum} -> [w230]
    tunnel: [w228] -> w4 mode=indexing
    shift-right: [w227] -> _
    shift-left: _ -> [w226]
    tunnel: [w224] -> w1
    tunnel: [w223] -> w5 mode=indexing
    stop <- w225 stop-if-true
    # "Gyro"
    n77 = Dequeue Element(queue=w235, error in (no error)=w234) -> (queue out=w232:refnum<queue>, element=w231:T20, error out=w233:errorcluster)  [unwired: 1 in, 1 out]
    n78 = case shown="No Error" w233 {
      selector: w233 -> [w239 w291]
      tunnel: w232 -> [w238 _]
      tunnel: w231 -> [w243 _]
      tunnel: [w237 TRUE] -> w225
      tunnel: w230 -> [w241 w292]
      tunnel: [w240 w292] -> w229
      tunnel: [w236 w291] -> w224
      frame No Error {
        n79 = Unbundle(w243) -> ("CMD"=w242:string)  [unwired: 1 out]
        n80 = case shown="\"GyroBoardAccess\"" w242 {
          tunnel: [w245 w251 w256 w269 w284 w286] -> w240
          tunnel: w241 -> [w245 w252 w253 w279 w284 w286]
          tunnel: w239 -> [w244 w247 w259 _ w283 w290]
          tunnel: [w244 w247 w257 w275 w283 w287] -> w236
          tunnel: w238 -> [_ _ w266 w278 _ w288]
          frame Default {
          }
          frame "Idle" {
            # "圖表歸零"
            n81 = property on="實際角度Chart" class="WFChart (strict)"("History Data"=cluster{"X":dbl, "Y":dbl}[] []) -> ()  [unwired: 2 in, 2 out]
            n82 = Bundle By Name(cluster=w252, "COM Port"="Serial Port", "baud rate"="baud rate", "Byte bits"="Byte bits") -> (w251:T12)
          }
          frame "GyroLink" {
            n83 = Format Date/Time String(time format string (%c)="%Y %m %d %H %M ") -> (date/time string=w264:string)  [unwired: 2 in]
            n84 = Concatenate Strings(w264, "GYro Angle.txt" ("element")) -> (w261:string)
            n85 = Enqueue Element(queue=w266, element=T20 {"CMD"="GyroBoardAccess", "DATA"=variant}, error in (no error)=w259) -> (error out=w258:errorcluster)  [unwired: 1 in, 2 out]
            n86 = Build Path(base path=path "C:/Users/baby3/OneDrive/Desktop/碩論/陀螺儀監控平台控制/GyroData", name or relative path=w261) -> (appended path=w260:path)
            n87 = Open/Create/Replace File(file path (use dialog)=w260, error in=w258, operation (0:open)=T21."replace or create") -> (refnum out=w255:refnum<file>, error out=w257:errorcluster)  [unwired: 3 in, 1 out]
            n88 = Bundle By Name(cluster=w253, "Save Path"=w255) -> (w256:T12)
          }
          frame "GyroBoardAccess" {
            n89 = Unbundle By Name(w279) -> ("COM Port"=w272:refnum<visa-resource-name>)
            n90 = call-poly "VISA Configure Serial Port"("VISA resource name"=w272, "baud rate (9600)"=u32 115200, "data bits (8)"=u16 8) -> ("VISA resource name out"=w271:refnum<visa-resource-name>, "error out"=w270:errorcluster)  [unwired: 11 in]
            n91 = VISA Read(VISA resource name=w271, byte count=u32 13, error in (no error)=w270) -> (read buffer=w282:string, error out=w281:errorcluster)  [unwired: 2 out]
            n92 = call "Arduino角度.vi"("error in"=w281, "read buffer"=w282) -> ("error out"=w276:errorcluster, "Waveform Chart"=w268:cluster{dbl, dbl})  [unwired: 2 in]
            "實際角度" <- w268
            "實際角度Chart" <- w268
            n93 = Enqueue Element(queue=w278, element=T20 {"CMD"="GyroBoardAccess", "DATA"=variant}, error in (no error)=w276) -> (error out=w275:errorcluster)  [unwired: 1 in, 2 out]
            n94 = Bundle By Name(cluster=w279, "實際角度"=w268) -> (w269:T12)
          }
          frame "GyroPanelUpdate" {
            n95 = Unbundle By Name(w284) -> ()  [unwired: 1 out]
          }
          frame "CloseBoard" {
            n96 = Unbundle By Name(w286) -> ("COM Port"=w285:refnum<visa-resource-name>)
            n97 = Flush Queue(queue=w288, error in (no error)=w290) -> (error out=w289:errorcluster)  [unwired: 2 out]
            n98 = VISA Close(VISA resource name=w285, error in (no error)=w289) -> (error out=w287:errorcluster)
          }
        }
        n99 = Unbundle By Name(w236) -> ("status"=w237:bool)
      }
      frame Error {
      }
    }
    n100 = Unbundle By Name(w229) -> ("實際角度"=w228:cluster{"A":dbl, "B":dbl})
    n101 = Tick Count (ms)() -> (millisecond timer value=w227:u32)
    n102 = Subtract(x=w227, y=w226) -> (x-y=w223:u32)
    "Gyro\nPeriod" <- w223
  }
  "error IO 2" <- w1
  n103 = Enqueue Element(queue=w20, element=T20 {"CMD"="Idle", "DATA"=variant}, error in (no error)=w23) -> (error out=w22:errorcluster)  [unwired: 1 in, 2 out]
  n104 = while {
    shift-right: [w296] -> w34
    shift-left: w22 -> [w299]
    tunnel: w21 -> [w300]
    tunnel: w20 -> [w294]
    stop <- w297 stop-if-true
    # "EventLoop"
    n105 = event shown="[7] \"ZABStop\", \"ZAB Start\": Value Change" {
      selector: _ -> [_ _ _ _ _ _ _ _ _ _ _ _]
      dyn-events: _ -> [_ _ _ _ _ _ _ _ _ _ _ _]
      timeout: _ -> [_ _ _ _ _ _ _ _ _ _ _ _]
      tunnel: w300 -> [w304 w308 w312 w319 w323 w327 w333 w337 _ _ w355 w358]
      tunnel: w299 -> [w303 w307 w311 w318 w322 w326 w332 w336 w343 w349 w354 w360]
      tunnel: [w302 w306 w310 w315 w321 w325 w331 w335 w342 w348 w352 w357] -> w296
      tunnel: [_ _ _ _ _ _ _ _ _ _ _ w362] -> w298
      tunnel: w294 -> [_ _ _ w313 _ _ _ _ w340 w346 w350 w361]
      event "Modbus Number of Inputs", "Serial Port", "TCP slave port", "baud rate", "Byte bits", "Modbus Address Starting": Value Change {
        n106 = event-data() -> ()  [unwired: 1 in, 1 out]
        n107 = Enqueue Element(queue=w304, element=T20 {"CMD"="SettingChange", "DATA"=variant}, error in (no error)=w303) -> (error out=w302:errorcluster)  [unwired: 1 in, 2 out]
      }
      event "Forward Enable?", "Reverse Enable?", "Motion Operation Mode", "Target Position (0)", "Acceleration (100000)", "Velocity (10000)", "Deacceleration (100000)", "Servo on": Value Change {
        n108 = event-data() -> ()  [unwired: 1 in, 1 out]
        n109 = Enqueue Element(queue=w308, element=T20 {"CMD"="ServoSetting", "DATA"=variant}, error in (no error)=w307) -> (error out=w306:errorcluster)  [unwired: 1 in, 2 out]
      }
      event "Z", "A", "B": Value Change {
        n110 = event-data() -> ()  [unwired: 1 in, 2 out]
        n111 = Enqueue Element(queue=w312, element=T20 {"CMD"="PIDSetting", "DATA"=variant}, error in (no error)=w311) -> (error out=w310:errorcluster)  [unwired: 1 in, 2 out]
      }
      event "Connect": Value Change {
        n112 = event-data() -> ()  [unwired: 1 in, 1 out]
        n113 = Enqueue Element(queue=w319, element=T20 {"CMD"="LinkBoard", "DATA"=variant}, error in (no error)=w318) -> (error out=w316:errorcluster)  [unwired: 1 in, 2 out]
        n114 = Enqueue Element(queue=w313, element=T20 {"CMD"="GyroLink", "DATA"=variant}, error in (no error)=w316) -> (error out=w315:errorcluster)  [unwired: 1 in, 2 out]
      }
      event "ServoButtonControl.AlarmReset": Value Change {
        n115 = event-data() -> ()  [unwired: 1 in, 1 out]
        n116 = Enqueue Element(queue=w323, element=T20 {"CMD"="AlarmReset", "DATA"=variant}, error in (no error)=w322) -> (error out=w321:errorcluster)  [unwired: 1 in, 2 out]
      }
      event "ServoButtonControl.Reset Encoder Position": Value Change {
        n117 = event-data() -> ()  [unwired: 1 in, 1 out]
        n118 = Enqueue Element(queue=w327, element=T20 {"CMD"="EncoderReset", "DATA"=variant}, error in (no error)=w326) -> (error out=w325:errorcluster)  [unwired: 1 in, 2 out]
      }
      event "ServoButtonControl": Value Change {
        n119 = event-data() -> ()  [unwired: 1 in, 1 out]
        n120 = Bundle By Name(cluster=T20 {"CMD"="Shooting", "DATA"=variant} ("element"), "DATA"="ServoButtonControl") -> (w329:T20)
        n121 = Enqueue Element(queue=w333, element=w329, error in (no error)=w332) -> (error out=w331:errorcluster)  [unwired: 1 in, 2 out]
      }
      event "ZABStop", "ZAB Start": Value Change {
        n122 = event-data() -> ()  [unwired: 1 in, 2 out]
        n123 = Enqueue Element(queue=w337, element=T20 {"CMD"="ZABMove", "DATA"=variant}, error in (no error)=w336) -> (error out=w335:errorcluster)  [unwired: 1 in, 2 out]
      }
      event "TimerON": Value Change {
        n124 = event-data() -> ("NewVal"=w338:bool)  [unwired: 1 in]
        n125 = Bundle By Name(cluster=T20 {"CMD"="ChangeTimerState", "DATA"=variant} ("element"), "DATA"=w338) -> (w339:T20)
        n126 = Enqueue Element(queue=w340, element=w339, error in (no error)=w343) -> (error out=w342:errorcluster)  [unwired: 1 in, 2 out]
      }
      event "Timer(ms)": Value Change {
        n127 = event-data() -> ("NewVal"=w344:i32)  [unwired: 1 in]
        n128 = Bundle By Name(cluster=T20 {"CMD"="ChangeTimerCount", "DATA"=variant} ("element"), "DATA"=w344) -> (w345:T20)
        n129 = Enqueue Element(queue=w346, element=w345, error in (no error)=w349) -> (error out=w348:errorcluster)  [unwired: 1 in, 2 out]
      }
      event "Close": Value Change {
        w351 = T20 {"CMD"="CloseBoard", "DATA"=variant} ("element")
        n130 = event-data() -> ()  [unwired: 1 in, 1 out]
        n131 = Enqueue Element At Opposite End(queue=w355, element=w351, error in (no error)=w354) -> (error out=w353:errorcluster)  [unwired: 1 in, 2 out]
        n132 = Enqueue Element At Opposite End(queue=w350, element=w351, error in (no error)=w353) -> (error out=w352:errorcluster)  [unwired: 1 in, 2 out]
      }
      event Panel Close? {
        w356 = T20 {"CMD"="CloseBoard", "DATA"=variant} ("element")
        w362 = TRUE
        n133 = event-data() -> ()  [unwired: 1 in, 1 out]
        n134 = Enqueue Element At Opposite End(queue=w361, element=w356, error in (no error)=w360) -> (error out=w359:errorcluster)  [unwired: 1 in, 2 out]
        n135 = event-data("Discard?"=w362) -> ()  [unwired: 1 in, 1 out]
        n136 = Enqueue Element At Opposite End(queue=w358, element=w356, error in (no error)=w359) -> (error out=w357:errorcluster)  [unwired: 1 in, 2 out]
      }
    }
    n137 = Unbundle By Name(w296) -> ("status"=w295:bool)
    n138 = Or(x=w295, y=w298) -> (x .or. y?=w297:bool)
  }
  n139 = Release Queue(queue=w20, error in (no error)=w34) -> (error out=w24:errorcluster)  [unwired: 1 in, 2 out]
  n140 = Release Queue(queue=w21, error in (no error)=w24) -> ()  [unwired: 1 in, 3 out]
  n141 = Unbundle By Name(w11) -> ("Save Path"=w10:refnum<file>)
  n142 = Unbundle By Name(w13) -> ("Save Path"=w12:refnum<file>)
  n143 = for {
    tunnel: [w372] -> w3 mode=indexing
    tunnel: w4 -> [w371] mode=indexing
    tunnel: w5 -> [w368] mode=indexing
    n144 = Unbundle(w371) -> ("A"=w370:dbl, "B"=w369:dbl)
    n145 = Format Into String(w370) -> (resulting string=w365:string)  [unwired: 3 in, 1 out]
    n146 = Format Into String(w369) -> (resulting string=w364:string)  [unwired: 3 in, 1 out]
    n147 = Format Into String(w368) -> (resulting string=w367:string)  [unwired: 3 in, 1 out]
    n148 = Insert Into Array(array=string[] ["Gyro Period(ms)："], new element #1=w367, new element #2="A：", new element #3=w365, new element #4="B：", new element #5=w364) -> (w372:string[])  [unwired: 1 in]
  }
  n149 = for {
    tunnel: [w383] -> w14 mode=indexing
    tunnel: w16 -> [w382] mode=indexing
    tunnel: w15 -> [w379] mode=indexing
    n150 = Unbundle(w382) -> ("A"=w381:dbl, "B"=w380:dbl)
    n151 = Format Into String(w381) -> (resulting string=w376:string)  [unwired: 3 in, 1 out]
    n152 = Format Into String(w380) -> (resulting string=w374:string)  [unwired: 3 in, 1 out]
    n153 = Format Into String(w379) -> (resulting string=w378:string)  [unwired: 3 in, 1 out]
    n154 = Insert Into Array(array=string[] ["Program Period(ms)："], new element #1=w378, new element #2="A：", new element #3=w376, new element #4="B：", new element #5=w374) -> (w383:string[])  [unwired: 1 in]
  }
  n155 = for {
    shift-right: [w387] -> w8
    shift-left: w10 -> [w389]
    shift-right: [w388] -> w9
    shift-left: _ -> [w386]
    tunnel: w3 -> [w385] mode=indexing
    n156 = Array To Spreadsheet String(delimiter (Tab)="\t", array=w385, 3:"%f" ("format string")) -> (spreadsheet string=w390:string)
    n157 = Write to Text File(file (use dialog)=w389, text=w390, error in=w386) -> (refnum out=w387:refnum<file>, error out=w388:errorcluster)  [unwired: 1 in, 1 out]
  }
  n158 = for {
    tunnel: w14 -> [w395] mode=indexing
    shift-right: [w393] -> w6
    shift-left: w12 -> [w397]
    shift-right: [w394] -> w7
    shift-left: _ -> [w396]
    n159 = Array To Spreadsheet String(delimiter (Tab)="\t", array=w395, 3:"%f" ("format string")) -> (spreadsheet string=w398:string)
    n160 = Write to Text File(file (use dialog)=w397, text=w398, error in=w396) -> (refnum out=w393:refnum<file>, error out=w394:errorcluster)  [unwired: 1 in, 1 out]
  }
  n161 = Close File(refnum=w8, error in=w9) -> ()  [unwired: 2 out]
  n162 = Close File(refnum=w6, error in=w7) -> ()  [unwired: 2 out]
